vi "Disconnect.vi"(8 "error in (no error)":errorcluster, 11 "Bobcat 640 in":refnum<class "Bobcat 640.lvclass">) -> (0 "error out":errorcluster, 3 "Bobcat 640 out":refnum<class "Bobcat 640.lvclass">)   [LabVIEW 2018, in "Bobcat 640.lvlib" / "Bobcat 640.lvclass"]
uses:
  Bobcat 640.lvclass
  Bobcat 640.lvclass/Bobcat 640.ctl
  <vilib>/vision/driver/NI_Vision_Acquisition_Software.lvlib
  PPLs/Camera/Parent/Camera.lvlibp/Camera.lvclass
  C:/AME Test Engineering/LabVIEW/PPLs/Camera/Parent/Camera.lvlibp/Camera.lvclass
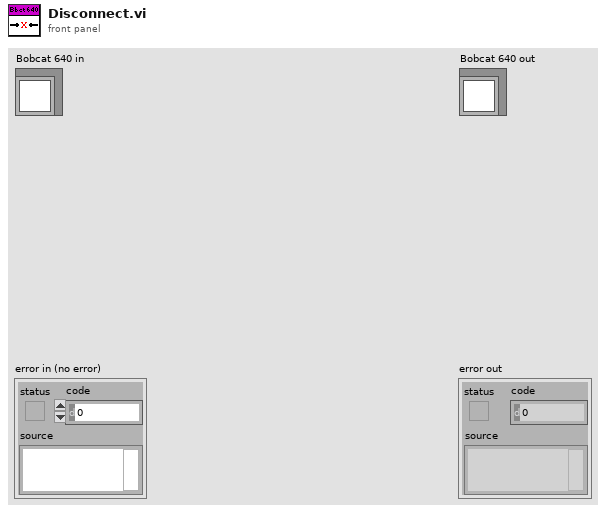
[diagram p1: front panel]
types:
  T1 = typedef "IMAQdx.ctl" = refnum<k21>
  T2 = typedef "Camera.lvlibp/IMAQ Image.ctl" = refnum<image>
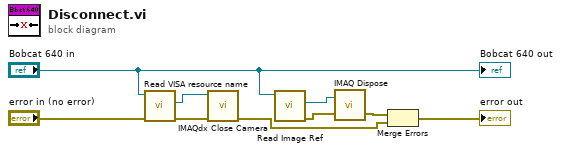
[diagram p0: block diagram]
diagram:
  n1 = call "Read VISA resource name.vi"("error in (no error)"="error in (no error)", "Bobcat 640 in"="Bobcat 640 in") -> ("error out"=w8:errorcluster, "IMAQdx Session"=w7:T1)  [unwired: 7 in, 1 out]
  n2 = call <vilib>:"IMAQdx Close Camera.vi"("error in"=w8, "Session In"=w7) -> ("error out"=w2:errorcluster)  [unwired: 9 in]
  n3 = call "Read Image Ref.vi"("Camera in"="Bobcat 640 in") -> ("error out"=w5:errorcluster, "Image"=w4:T2)  [unwired: 8 in, 1 out]
  n4 = call "IMAQ Dispose"("Image"=w4, "error in (no error)"=w5) -> ("error out"=w3:errorcluster)  [unwired: 4 in]
  n5 = Merge Errors(w3, w2) -> (→"error out":errorcluster)
  "Bobcat 640 out" <- "Bobcat 640 in"
